vi "子VI对话框.vi"() -> ()   [LabVIEW 2018]
panel:
  out "登陆结果":string
  in  "密码":string
  in  "用户名":string
  in  "退出":bool
  in  "登录":bool
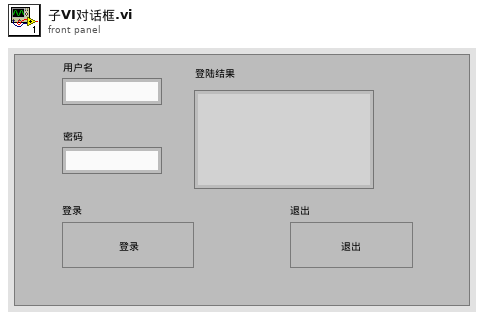
[diagram p1: front panel]
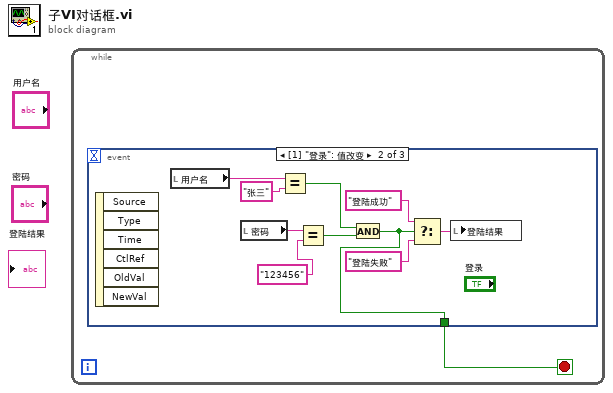
[diagram p0: block diagram]
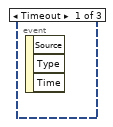
[diagram p2: hidden frame]
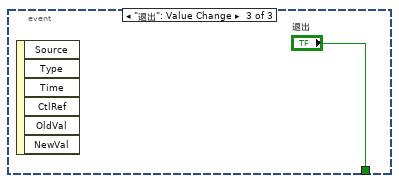
[diagram p3: hidden frame]
diagram:
  n1 = while {
    stop <- w1 stop-if-true
    n2 = event shown="[1] \"登录\": 值改变" {
      selector: _ -> [_ _ _]
      dyn-events: _ -> [_ _ _]
      timeout: _ -> [_ _ _]
      tunnel: [_ w2 "退出"] -> w1
      event Timeout {
        n3 = event-data() -> ()  [unwired: 1 in, 3 out]
      }
      event "登录": Value Change {
        n4 = event-data() -> ()  [unwired: 1 in, 6 out]
        n5 = local read "用户名"() -> (w8:string)
        n6 = local read "密码"() -> (w7:string)
        n7 = Equal?(x=w8, y="张三") -> (x = y?=w11:bool)
        n8 = Equal?(x=w7, y="123456") -> (x = y?=w10:bool)
        n9 = And(x=w11, y=w10) -> (x .and. y?=w2:bool)
        n10 = Select(t="登陆成功" ("y"), s=w2, f="登陆失败" ("y")) -> (s? t:f=w4:string)
        n11 = local write "登陆结果"(w4) -> ()
      }
      event "退出": Value Change {
        n12 = event-data() -> ()  [unwired: 1 in, 6 out]
      }
    }
  }
